vi "Decode DM Normal.vi"(11 "DataMatrix Text":string) -> (3 "DM CONTENT OUT":T1)   [LabVIEW 2024]
panel:
  out "Array":bool[](array[boolean])
  out "Character Array":string[](array[string])
  out "DM Data":string[](array[string])
  out "DM Order":string[](array[string])
  out "Sep":string
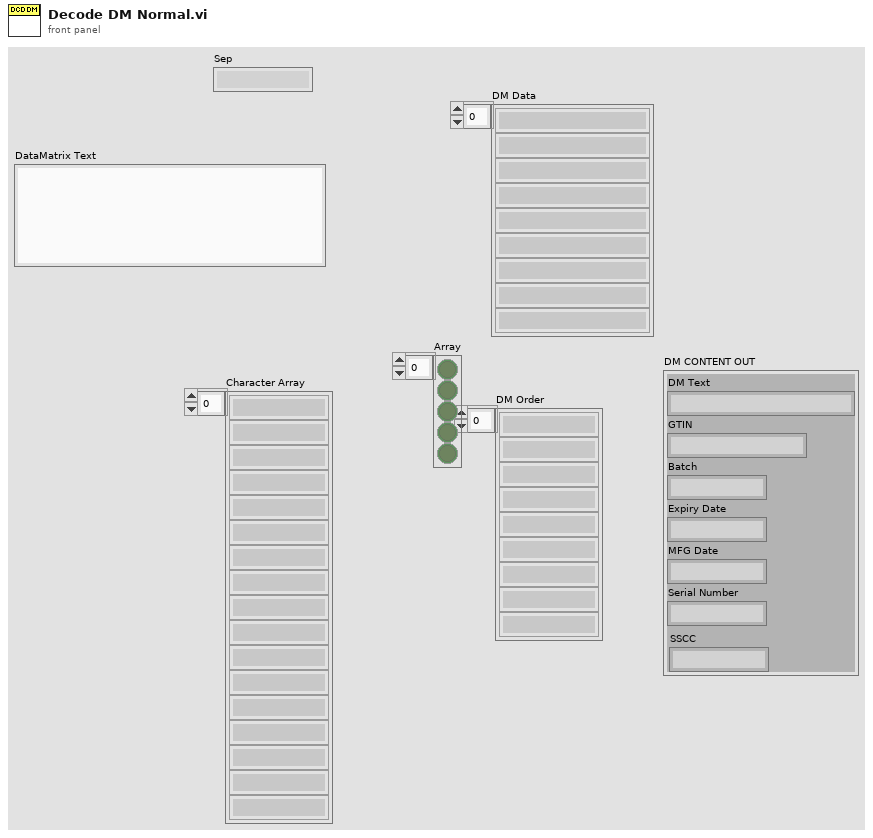
[diagram p1: front panel]
types:
  T1 = cluster{"DM Text":string, "GTIN":string, "Batch":string, "Expiry Date":string, "MFG Date":string, "Serial Number":string, "SSCC":string}
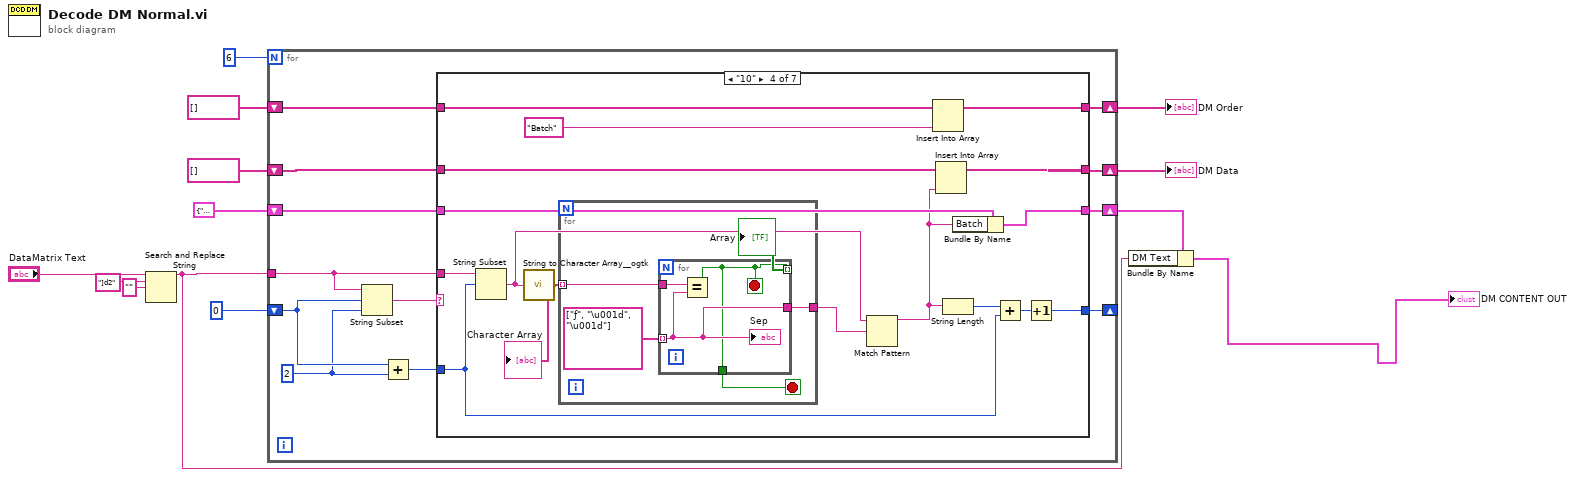
[diagram p0: block diagram]
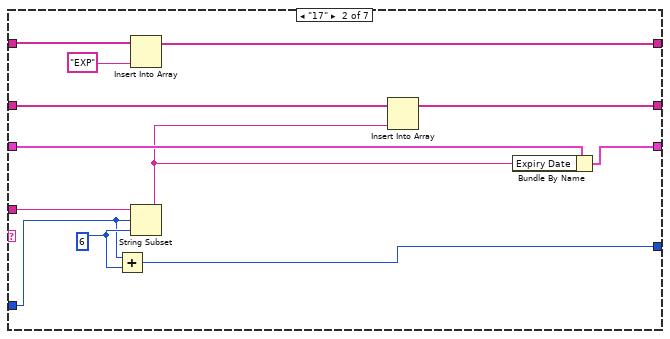
[diagram p3: hidden frame]
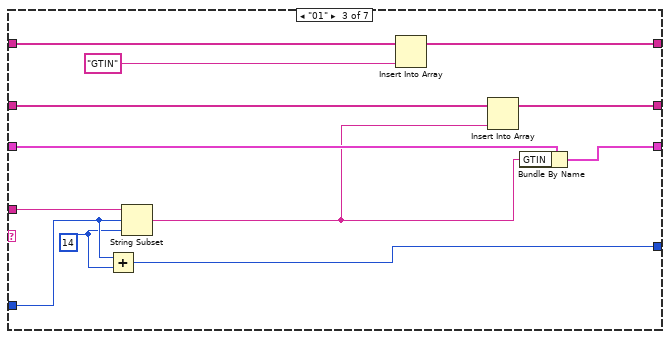
[diagram p4: hidden frame]
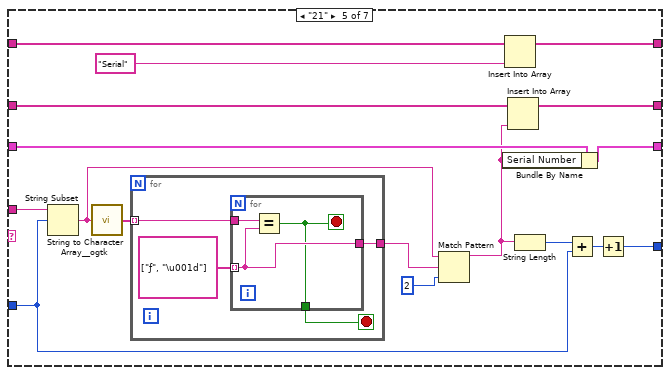
[diagram p5: hidden frame]
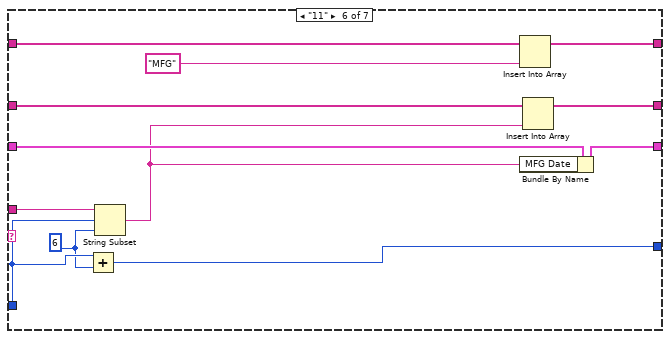
[diagram p6: hidden frame]
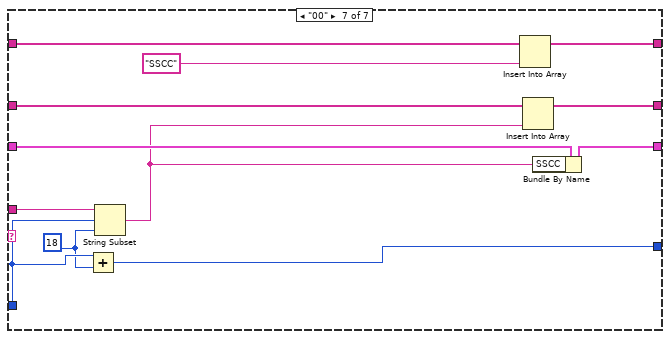
[diagram p7: hidden frame]
diagram:
  n1 = Search and Replace String(input string="DataMatrix Text", search string="]d2" ("input string"), replace string="" ("replace string (\"\")")) -> (result string=w4:string)  [unwired: 5 in, 3 out]
  n2 = for {
    N: 6 -> [_]
    tunnel: w4 -> [w23]
    shift-right: [w24] -> _
    shift-left: 0 -> [w22]
    shift-right: [w19] -> w10
    shift-left: string[] [] -> [w18]
    shift-right: [w17] -> w8
    shift-left: string[] [] -> [w16]
    shift-right: [w15] -> w7
    shift-left: T1 {"DM Text"="", "GTIN"="", "Batch"="", "Expiry Date"="", "MFG Date"="", "Serial Number"="", "SSCC"=""} ("DM CONTENT OUT") -> [w14]
    w21 = 2 ("length (rest)")
    n3 = String Subset(string=w23, offset (0)=w22, length (rest)=w21) -> (substring=w25:string)
    n4 = Add(x=w22, y=w21) -> (x+y=w20:i32)
    n5 = case shown="\"10\"" w25 {
      tunnel: w23 -> [_ w41 w53 w66 w91 w113 w125]
      tunnel: w20 -> [w27 w38 w52 w65 w90 w112 w124]
      tunnel: [w27 w39 w50 w67 w92 w110 w122] -> w24
      tunnel: [w29 w35 w47 w62 w87 w107 w119] -> w19
      tunnel: w18 -> [w29 w36 w48 w63 w88 w108 w120]
      tunnel: [w28 w33 w46 w61 w86 w105 w117] -> w17
      tunnel: w16 -> [w28 w34 w45 w60 w85 w106 w118]
      tunnel: [w26 w31 w43 w58 w83 w103 w115] -> w15
      tunnel: w14 -> [w26 w32 w44 w59 w84 w104 w116]
      frame Default {
      }
      frame "17" {
        w40 = 6 ("length (rest)")
        n6 = Add(x=w38, y=w40) -> (x+y=w39:i32)
        n7 = Insert Into Array(array=w36, new element="EXP" ("regular expression")) -> (w35:string[])  [unwired: 1 in]
        n8 = String Subset(string=w41, offset (0)=w38, length (rest)=w40) -> (substring=w30:string)
        n9 = Insert Into Array(array=w34, new element=w30) -> (w33:string[])  [unwired: 1 in]
        n10 = Bundle By Name(cluster=w32, "Expiry Date"=w30) -> (w31:T1)
      }
      frame "01" {
        w51 = 14 ("length (rest)")
        n11 = Add(x=w52, y=w51) -> (x+y=w50:i32)
        n12 = String Subset(string=w53, offset (0)=w52, length (rest)=w51) -> (substring=w42:string)
        n13 = Insert Into Array(array=w48, new element="GTIN" ("regular expression")) -> (w47:string[])  [unwired: 1 in]
        n14 = Insert Into Array(array=w45, new element=w42) -> (w46:string[])  [unwired: 1 in]
        n15 = Bundle By Name(cluster=w44, "GTIN"=w42) -> (w43:T1)
      }
      frame "10" {
        n16 = String Subset(string=w66, offset (0)=w65) -> (substring=w55:string)  [unwired: 1 in]
        n17 = call "String to Character Array__ogtk.vi"("Input String"=w55) -> ("Character Array"=w57:string[])
        "Character Array" <- w57
        n18 = for {
          tunnel: w57 -> [w73] mode=indexing
          tunnel: [w72] -> w56
          stop <- w71 stop-if-true
          n19 = for {
            tunnel: string[] ["ƒ", "\u001d", "\u001d"] -> [w76] mode=indexing
            tunnel: w73 -> [w77]
            tunnel: [w76] -> w72
            tunnel: [w75] -> w71
            tunnel: [w75] -> w70 mode=indexing
            stop <- w75 stop-if-true
            n20 = Equal?(x=w77, y=w76) -> (x = y?=w75:bool)
            "Sep" <- w76
          }
          "Array" <- w70
        }
        n21 = Match Pattern(string=w55, regular expression=w56) -> (before substring=w54:string)  [unwired: 1 in, 3 out]
        n22 = Insert Into Array(array=w63, new element="Batch" ("regular expression")) -> (w62:string[])  [unwired: 1 in]
        n23 = Insert Into Array(array=w60, new element=w54) -> (w61:string[])  [unwired: 1 in]
        n24 = String Length(string=w54) -> (length=w68:i32)
        n25 = Bundle By Name(cluster=w59, "Batch"=w54) -> (w58:T1)
        n26 = Add(x=w68, y=w65) -> (x+y=w69:i32)
        n27 = Increment(x=w69) -> (x+1=w67:i32)
      }
      frame "21" {
        n28 = String Subset(string=w91, offset (0)=w90) -> (substring=w79:string)  [unwired: 1 in]
        n29 = call "String to Character Array__ogtk.vi"("Input String"=w79) -> ("Character Array"=w82:string[])
        n30 = for {
          tunnel: w82 -> [w97] mode=indexing
          tunnel: [w96] -> w80
          stop <- w95 stop-if-true
          n31 = for {
            tunnel: string[] ["ƒ", "\u001d"] -> [w100] mode=indexing
            tunnel: w97 -> [w101]
            tunnel: [w100] -> w96
            tunnel: [w99] -> w95
            stop <- w99 stop-if-true
            n32 = Equal?(x=w101, y=w100) -> (x = y?=w99:bool)
          }
        }
        n33 = Match Pattern(string=w79, regular expression=w80, offset (0)=2) -> (before substring=w78:string)  [unwired: 3 out]
        n34 = Bundle By Name(cluster=w84, "Serial Number"=w78) -> (w83:T1)
        n35 = Insert Into Array(array=w88, new element="Serial" ("regular expression")) -> (w87:string[])  [unwired: 1 in]
        n36 = Insert Into Array(array=w85, new element=w78) -> (w86:string[])  [unwired: 1 in]
        n37 = String Length(string=w78) -> (length=w93:i32)
        n38 = Add(x=w93, y=w90) -> (x+y=w94:i32)
        n39 = Increment(x=w94) -> (x+1=w92:i32)
      }
      frame "11" {
        w111 = 6 ("length (rest)")
        n40 = Add(x=w112, y=w111) -> (x+y=w110:i32)
        n41 = String Subset(string=w113, offset (0)=w112, length (rest)=w111) -> (substring=w102:string)
        n42 = Insert Into Array(array=w108, new element="MFG" ("regular expression")) -> (w107:string[])  [unwired: 1 in]
        n43 = Bundle By Name(cluster=w104, "MFG Date"=w102) -> (w103:T1)
        n44 = Insert Into Array(array=w106, new element=w102) -> (w105:string[])  [unwired: 1 in]
      }
      frame "00" {
        w123 = 18 ("length (rest)")
        n45 = Add(x=w124, y=w123) -> (x+y=w122:i32)
        n46 = String Subset(string=w125, offset (0)=w124, length (rest)=w123) -> (substring=w114:string)
        n47 = Insert Into Array(array=w120, new element="SSCC" ("regular expression")) -> (w119:string[])  [unwired: 1 in]
        n48 = Insert Into Array(array=w118, new element=w114) -> (w117:string[])  [unwired: 1 in]
        n49 = Bundle By Name(cluster=w116, "SSCC"=w114) -> (w115:T1)
      }
    }
  }
  "DM Order" <- w10
  "DM Data" <- w8
  n50 = Bundle By Name(cluster=w7, "DM Text"=w4) -> (→"DM CONTENT OUT":T1)
